vi "send_go.vi"   [LabVIEW 2014]
uses:
  g_ECS02_Command.vi
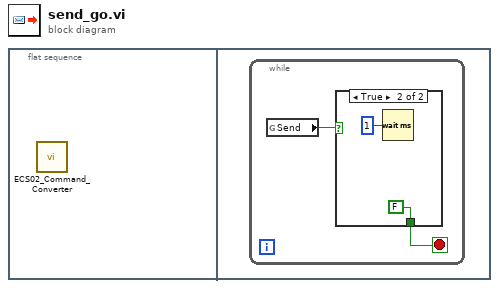
[diagram p0: block diagram]
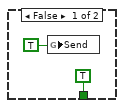
[diagram p2: hidden frame]
diagram:
  n1 = flat-sequence {
    frame #0 {
      n2 = call "ECS02_Command_Converter.vi"() -> ()  [unwired: 12 in]
    }
    frame #1 {
      n3 = while {
        stop <- w1 stop-if-true
        n4 = global read "g_ECS02_Command.vi" "Send"() -> (w2:bool)
        n5 = case shown="True" w2 {
          tunnel: [TRUE FALSE] -> w1
          frame False {
            n6 = global write "g_ECS02_Command.vi" "Send"(TRUE ("Send")) -> ()
          }
          frame True {
            n7 = Wait (ms)(milliseconds to wait=u32 1) -> ()  [unwired: 1 out]
          }
        }
      }
    }
  }
